vi "PolhemusConfigCoerceLF.vi"() -> ()   [LabVIEW 2009]
uses:
  BaudRateSelector.ctl
  <vilib>/Instr/_visa.llb/VISA Configure Serial Port (Instr).vi
panel:
  out "Output":string
  in  "Input":string="P"
  in  "Test Configuration?":bool
  in  "Only Send Custom\n(Save Feature still in effect)":bool
  in  "Special Commands":string
  in  "Station Controls":cluster{"Output Listing":u16[]}[](array[cluster])=[{"Output Listing"=[2, 4]}, {"Output Listing"=[2, 4, 1]}] {"Output Listing" items=["Cartesian Coordinates"=2, "Euler Orientation"=4, "ASCII Space"=0, "CR, LF"=1]}
  in  "Save to EEPROM?":bool
  in  "Output Format":enum16{"ASCII", "Binary"}(ring)=enum."Binary"
  in  "Units":enum16{"Inches", "Centimeters"}(ring)=enum."Centimeters"
  in  "Parity":enum16{"None", "Odd", "Even", "Mark", "Space"}(ring)
  in  "Data Bits":u16=8 min=7 max=8 step=1
  in  "Baud Rate":T1=115200 items=["1200"=1200, "2400"=2400, "4800"=4800, "9600"=9600, "19200"=19200, "38400"=38400, "57600"=57600, "115200"=115200]
  in  "VISA resource name":refnum<visa-resource-name>="COM3"
  # "Polhemus 3SPACE FASTRAK Configuration Tool\n~~~~~~~~~"
  # "Basic Serial Information"
  # "Polhemus Settings Config"
  # "Custom Commands to Send"
  # "This tool sends commands to the Polhemus Fastrak to configure it for desired use.\nIn addition to basic status configuration, the output of the receiver functions can be changed here. The 4 most basic commands are listed, however other commands can be issued by typing in the number specified by the manual on pg. 98 to the right of the menu.\nTo remove a command, right-click and select  \"Delete Element\"."
  # "If Data Bits = 8, Parity must be \"None\""
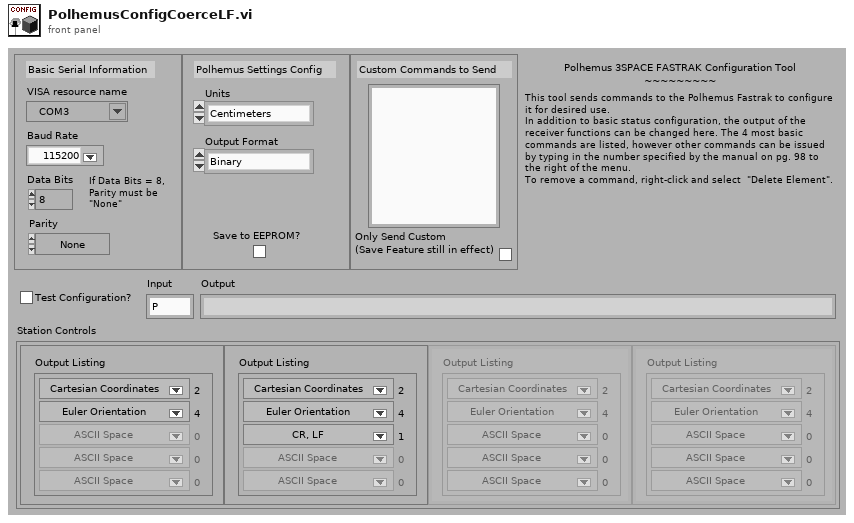
[diagram p1: front panel]
types:
  T1 = typedef "BaudRateSelector.ctl" = u32
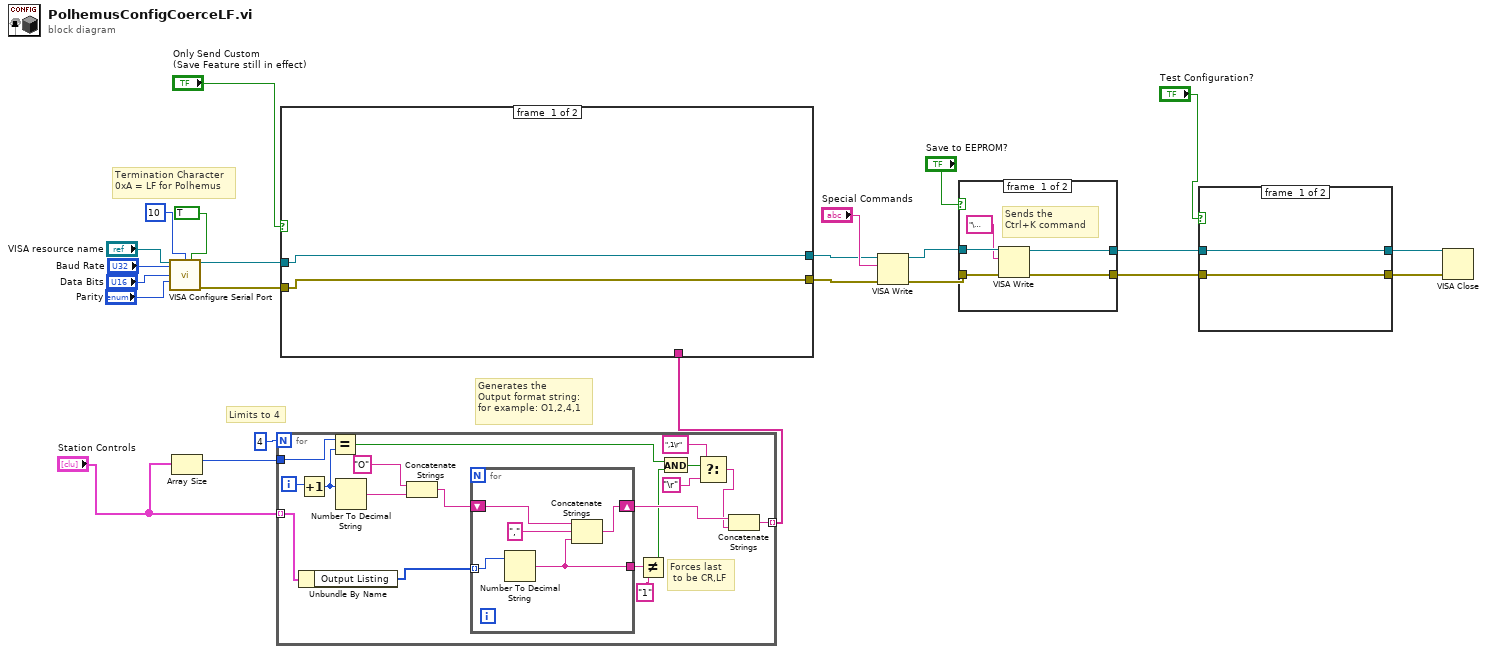
[diagram p0: block diagram]
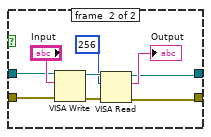
[diagram p2: hidden frame]
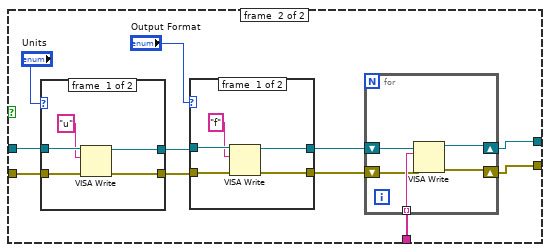
[diagram p3: hidden frame]
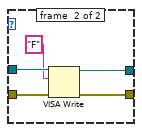
[diagram p4: hidden frame]
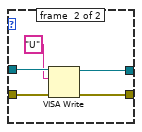
[diagram p5: hidden frame]
diagram:
  # "Limits to 4"
  # "Generates the\nOutput format string:\nfor example: O1,2,4,1"
  # "Termination Character\n0xA = LF for Polhemus"
  n1 = call-poly "VISA Configure Serial Port"("VISA resource name"="VISA resource name", "termination char\n(0xA = '\\n' = LF)"=u8 10 ("termination char\n(0xA = '\\n' = LF)"), "Enable Termination\nChar (T)"=TRUE ("Enable Termination\nChar (T)"), "baud rate (9600)"="Baud Rate", "data bits (8)"="Data Bits", "parity (0:none)"="Parity") -> ("VISA resource name out"=w18:refnum<visa-resource-name>, "error out"=w17:errorcluster)  [unwired: 8 in]
  n2 = Array Size(array="Station Controls") -> (size(s)=w1:i32)
  n3 = for {
    N: 4 -> [_]
    tunnel: "Station Controls" -> [w42] mode=indexing
    tunnel: [w37] -> w16 mode=indexing
    tunnel: w1 -> [w35]
    i -> [w36]
    # "Forces last\n to be CR,LF"
    n4 = Increment(x=w36) -> (x+1=w34:i32)
    n5 = Unbundle By Name(w42) -> ("Output Listing"=w33:u16[])
    n6 = Equal?(x=w35, y=w34) -> (x = y?=w30:bool)
    n7 = Number To Decimal String(number=w34) -> (decimal integer string=w40:string)  [unwired: 1 in]
    n8 = Concatenate Strings("O", w40) -> (w39:string)
    n9 = for {
      tunnel: w33 -> [w47] mode=indexing
      shift-right: [w44] -> w38
      shift-left: w39 -> [w46]
      tunnel: [w43] -> w32
      n10 = Number To Decimal String(number=w47) -> (decimal integer string=w43:string)  [unwired: 1 in]
      n11 = Concatenate Strings(w46, ",", w43) -> (w44:string)
    }
    n12 = Not Equal?(x=w32, y="1") -> (x != y?=w29:bool)
    n13 = And(x=w30, y=w29) -> (x .and. y?=w28:bool)
    n14 = Select(t=",1\r", s=w28, f="\r") -> (s? t:f=w25:string)
    n15 = Concatenate Strings(w38, w25) -> (w37:string)
  }
  n16 = case shown="False" "Only Send Custom\n(Save Feature still in effect)" {
    tunnel: w18 -> [w49 w59]
    tunnel: w17 -> [w48 w58]
    tunnel: w16 -> [_ w54]
    tunnel: [w49 w51] -> w13
    tunnel: [w48 w50] -> w11
    frame #0 {
    }
    frame #1 {
      n17 = case shown="\"Centimeters\", Default" "Units" {
        tunnel: w59 -> [w79 w84]
        tunnel: w58 -> [w80 w85]
        tunnel: [w77 w82] -> w56
        tunnel: [w76 w81] -> w55
        frame #0 {
          n18 = VISA Write(VISA resource name=w79, write buffer="u", error in (no error)=w80) -> (VISA resource name out=w77:refnum<visa-resource-name>, error out=w76:errorcluster)  [unwired: 1 out]
        }
        frame #1 {
          n19 = VISA Write(VISA resource name=w84, write buffer="U", error in (no error)=w85) -> (VISA resource name out=w82:refnum<visa-resource-name>, error out=w81:errorcluster)  [unwired: 1 out]
        }
      }
      n20 = case shown="\"Binary\", Default" "Output Format" {
        tunnel: w56 -> [w69 w74]
        tunnel: w55 -> [w70 w75]
        tunnel: [w67 w72] -> w52
        tunnel: [w66 w71] -> w53
        frame #0 {
          n21 = VISA Write(VISA resource name=w69, write buffer="f", error in (no error)=w70) -> (VISA resource name out=w67:refnum<visa-resource-name>, error out=w66:errorcluster)  [unwired: 1 out]
        }
        frame #1 {
          n22 = VISA Write(VISA resource name=w74, write buffer="F", error in (no error)=w75) -> (VISA resource name out=w72:refnum<visa-resource-name>, error out=w71:errorcluster)  [unwired: 1 out]
        }
      }
      n23 = for {
        tunnel: w54 -> [w65] mode=indexing
        shift-right: [w62] -> w51
        shift-left: w52 -> [w63]
        shift-right: [w61] -> w50
        shift-left: w53 -> [w64]
        n24 = VISA Write(VISA resource name=w63, write buffer=w65, error in (no error)=w64) -> (VISA resource name out=w62:refnum<visa-resource-name>, error out=w61:errorcluster)  [unwired: 1 out]
      }
    }
  }
  n25 = VISA Write(VISA resource name=w13, write buffer="Special Commands", error in (no error)=w11) -> (VISA resource name out=w12:refnum<visa-resource-name>, error out=w10:errorcluster)  [unwired: 1 out]
  n26 = case shown="True" "Save to EEPROM?" {
    tunnel: w12 -> [w89 w92]
    tunnel: w10 -> [w90 w91]
    tunnel: [w87 w92] -> w7
    tunnel: [w86 w91] -> w6
    frame #0 {
      # "Sends the\nCtrl+K command"
      n27 = VISA Write(VISA resource name=w89, write buffer="\u000b", error in (no error)=w90) -> (VISA resource name out=w87:refnum<visa-resource-name>, error out=w86:errorcluster)  [unwired: 1 out]
    }
    frame #1 {
    }
  }
  n28 = case shown="True" "Test Configuration?" {
    tunnel: w7 -> [w94 w102]
    tunnel: w6 -> [w93 w101]
    tunnel: [w94 w97] -> w5
    tunnel: [w93 w96] -> w4
    frame #0 {
    }
    frame #1 {
      n29 = VISA Write(VISA resource name=w102, write buffer="Input", error in (no error)=w101) -> (VISA resource name out=w100:refnum<visa-resource-name>, error out=w99:errorcluster)  [unwired: 1 out]
      n30 = VISA Read(VISA resource name=w100, byte count=u32 256, error in (no error)=w99) -> (VISA resource name out=w97:refnum<visa-resource-name>, read buffer=→"Output":string, error out=w96:errorcluster)  [unwired: 1 out]
    }
  }
  n31 = VISA Close(VISA resource name=w5, error in (no error)=w4) -> ()  [unwired: 1 out]
